vi "Istwerte verarbeiten Alarme.vi"(8 "error in (no error)":errorcluster caption="Fehler (Eingang, kein Fehler)", 10 "Istwerte":u16[](array[numeric]), 11 "mini8 Steuerung PNS Eingang":refnum<class "mini8 Steuerung PNS.lvclass">) -> (0 "error out":errorcluster caption="Fehler (Ausgang)", 3 "mini8 Steuerung PNS Ausgang":refnum<class "mini8 Steuerung PNS.lvclass">)   [LabVIEW 2020, in "mini8 Steuerung PNS.lvclass"]
uses:
  mini8 Steuerung PNS.lvclass
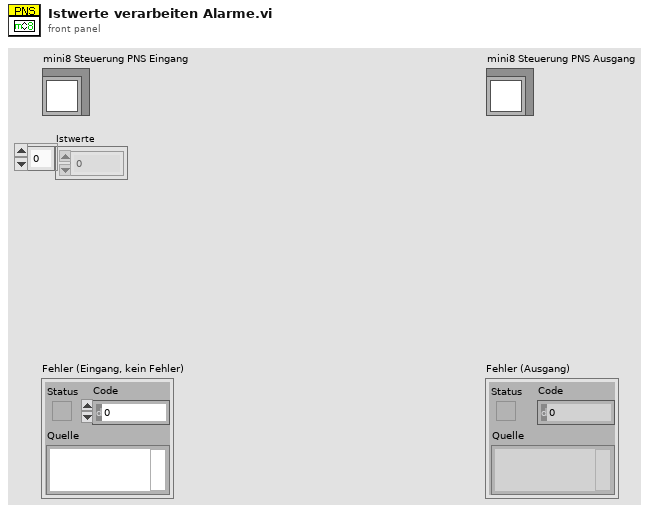
[diagram p1: front panel]
types:
  T1 = cluster{"[0]":u16, "[1]":u16, "[2]":u16, "[3]":u16, "[4]":u16, "[5]":u16, "[6]":u16, "[7]":u16, "[8]":u16, "[9]":u16, "[10]":u16, "[11]":u16, "[12]":u16, "[13]":u16, "[14]":u16, "[15]":u16}
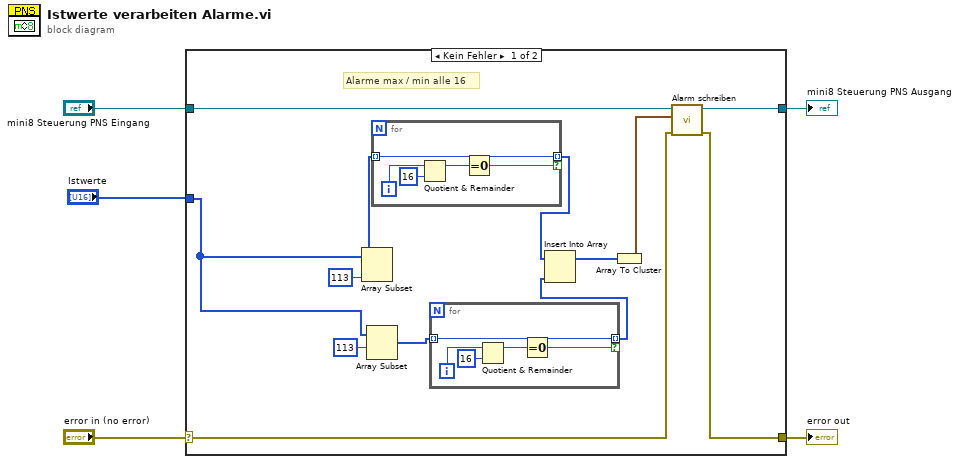
[diagram p0: block diagram]
diagram:
  n1 = case shown="Kein Fehler" "error in (no error)" {
    selector: "error in (no error)" -> [w7 w30]
    tunnel: [w6 w30] -> w4
    tunnel: [w8 w29] -> w2
    tunnel: "mini8 Steuerung PNS Eingang" -> [w18 w29]
    tunnel: "Istwerte" -> [w9 _]
    frame No Error {
      # "Alarme max / min alle 16"
      n2 = Array Subset(array=w9, length=113 ("Länge")) -> (w15:u16[])  [unwired: 1 in]
      n3 = Array Subset(array=w9, index=113 ("Index")) -> (w13:u16[])  [unwired: 1 in]
      n4 = for {
        tunnel: w15 -> [w28] mode=indexing
        tunnel: [w28] -> w12 mode=indexing if=w24
        i -> [w27]
        n5 = Quotient & Remainder(x=w27, y=16) -> (x-y*floor(x/y)=w25:i32)  [unwired: 1 out]
        n6 = Equal To 0?(x=w25) -> (x = 0?=w24:bool)
      }
      n7 = for {
        tunnel: w13 -> [w19] mode=indexing
        tunnel: [w19] -> w10 mode=indexing if=w20
        i -> [w23]
        n8 = Quotient & Remainder(x=w23, y=16) -> (x-y*floor(x/y)=w21:i32)  [unwired: 1 out]
        n9 = Equal To 0?(x=w21) -> (x = 0?=w20:bool)
      }
      n10 = Insert Into Array(array=w12, new element=w10) -> (w11:u16[])  [unwired: 1 in]
      n11 = Array To Cluster(array=w11) -> (cluster=w17:T1)
      n12 = call-dynamic "Alarm schreiben.vi"("error in (no error)"=w7, "Alarm"=w17, "Steuerung PNS (Eingang)"=w18) -> ("error out"=w6:errorcluster, "Steuerung PNS (Ausgang)"=w8:refnum<class "mini8 Steuerung PNS.lvclass">)  [unwired: 7 in]
    }
    frame Error {
    }
  }
  "error out" <- w4
  "mini8 Steuerung PNS Ausgang" <- w2
